vi "SMO.Control Experiment.Client.vi"(8 "error in (no error)":errorcluster, 9 "Data":variant, 10 "Command":T1, 11 "Sequence Experiment":refnum<class "SMO.Control Experiment.lvclass">) -> (0 "error out":errorcluster, 1 "Data out":variant, 2 "Command":string, 3 "Sequence Experiment out":refnum<class "SMO.Control Experiment.lvclass">)   [LabVIEW 2019, in "SMO.Control Experiment.lvclass"]
uses:
  SMO.Control Experiment.lvclass
  adaf5e02-75a0-4c77-8d0c-0d3e2c278268.vi
  Typedefs/SMO.Control Experiment.Commands--Enum.ctl
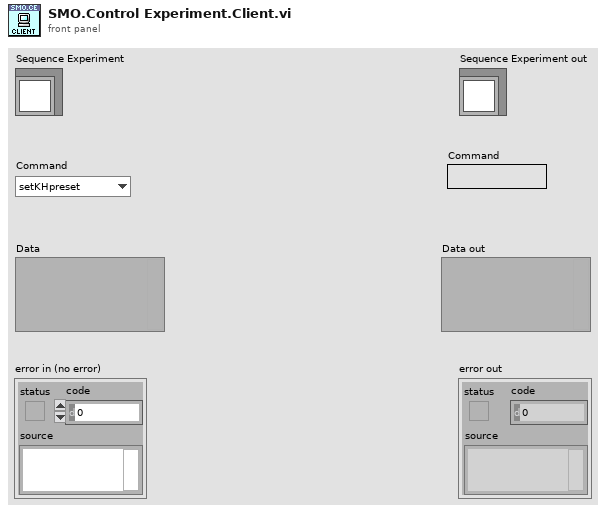
[diagram p1: front panel]
types:
  T1 = typedef "SMO.Control Experiment.lvclass/SMO.Control Experiment.Commands--Enum.ctl" = enum16{"setKHpreset", "getXML", "saveData"}
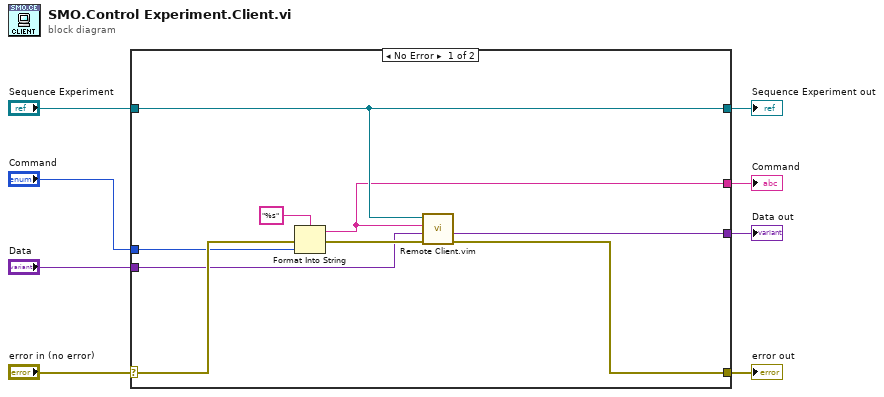
[diagram p0: block diagram]
diagram:
  n1 = case shown="No Error" "error in (no error)" {
    selector: "error in (no error)" -> [w14 w19]
    tunnel: [w13 w19] -> w7
    tunnel: [w17 w18] -> w5
    tunnel: "Sequence Experiment" -> [w17 w18]
    tunnel: "Data" -> [w9 _]
    tunnel: "Command" -> [w12 _]
    tunnel: [w11 _] -> w2
    tunnel: [w10 _] -> w1
    frame No Error {
      n2 = Format Into String(format string="%s", error in=w14, w12) -> (resulting string=w10:string, error out=w15:errorcluster)  [unwired: 1 in]
      n3 = call "Remote Client.vim"("error in (no error)"=w15, "params"=w9, "method"=w10, "Instrument in"=w17) -> ("error out"=w13:errorcluster, "Data out"=w11:variant)  [unwired: 4 in, 2 out]
    }
    frame Error {
    }
  }
  "error out" <- w7
  "Sequence Experiment out" <- w5
  "Data out" <- w2
  "Command" <- w1
